vi "Configure Math.vi"   [LabVIEW 2009, in "Agilent 8000 Series.lvlib"]
doc: "Configure the Math Operation"
uses:
  Agilent 8000 Series.lvlib
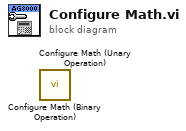
[diagram p0: block diagram]
diagram:
  n1 = call "Configure Math (Binary Operation).vi"() -> ()  [unwired: 14 in, 2 out]
  n2 = call "Configure Math (Unary Operation).vi"() -> ()  [unwired: 14 in, 2 out]
